vi "Build Dqmh Module Relationship Sub Graph.vi"(7 "Link Type":T1, 9 "Module Name":string, 10 "Links Info":T4[](array[typedef]), 11 "Graph in":refnum<class "Graph.lvclass">) -> (1 "Specific Edge Shape":T2[](array[typedef]), 2 "Specific Node Shape":T3[](array[typedef]), 3 "Graph out":refnum<class "Graph.lvclass">)   [LabVIEW 2021, in "TAF Proj Document Type.lvlib" / "Dqmh Module.lvclass"]
uses:
  <vilib>/Wovalab/AntiDoc/Document Type/Add-ons/LabVIEW TAF Project/Dqmh Module/Dqmh Module.lvclass
  <vilib>/Wovalab/AntiDoc/Document Type/Add-ons/LabVIEW TAF Project/Dqmh Module/Event Callers--cluster.ctl
  <vilib>/Wovalab/AntiDoc/GraphBuilder/Graph/Graph.lvclass
  <vilib>/Wovalab/AntiDoc/GraphBuilder/Renderer/Graphviz/Specific Node Shape Def.ctl
  <vilib>/Wovalab/AntiDoc/GraphBuilder/Shapes/Node/Graphviz/Graphviz Node Shape.lvclass
  <vilib>/Wovalab/AntiDoc/GraphBuilder/Renderer/Graphviz/Specific Edge Shape Def.ctl
  <vilib>/Wovalab/AntiDoc/GraphBuilder/Shapes/Edge/Graphviz/Graphviz Edge Shape.lvclass
  <vilib>/Wovalab/AntiDoc/Document Type/Add-ons/LabVIEW TAF Project/Dqmh Module/Link Type--enum.ctl
  <vilib>/Wovalab/AntiDoc/Document Type/Add-ons/LabVIEW TAF Project/Shared/Dqmh Event Module Link Type.ctl
  <vilib>/Wovalab/AntiDoc/Document Type/Add-ons/LabVIEW TAF Project/TAF Proj Document Type.lvlib
  <vilib>/Wovalab/AntiDoc/GraphBuilder/Renderer/Graphviz/Graphviz.lvclass
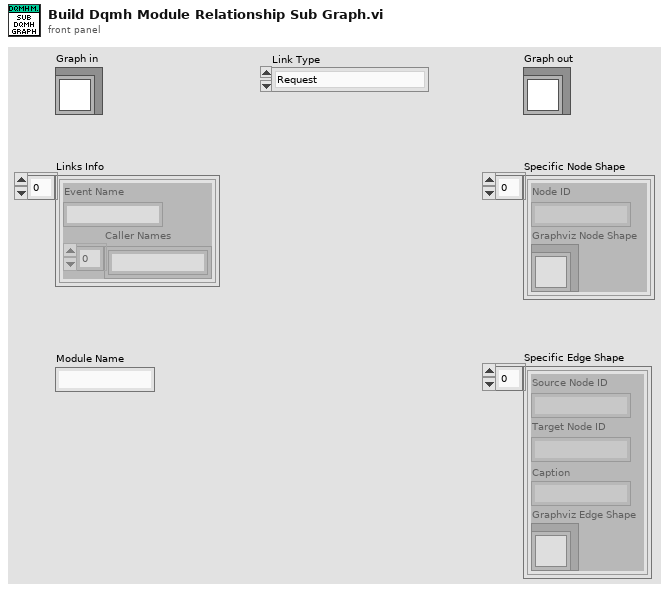
[diagram p1: front panel]
types:
  T1 = typedef "TAF Proj Document Type.lvlib/Dqmh Module.lvclass/Link Type--enum.ctl" = enum16{"Request", "Request With Reply", "Broadcast", "Registred Broadcast", "Used Requests", "Used Requests With Reply"}
  T2 = typedef "GraphBuilder.lvlib/Graphviz.lvclass/Specific Edge Shape Def.ctl" = cluster{"Source Node ID":string, "Target Node ID":string, "Caption":string, "Graphviz Edge Shape":refnum<class "Graphviz Edge Shape.lvclass">}
  T3 = typedef "GraphBuilder.lvlib/Graphviz.lvclass/Specific Node Shape Def.ctl" = cluster{"Node ID":string, "Graphviz Node Shape":refnum<class "Graphviz Node Shape.lvclass">}
  T4 = typedef "TAF Proj Document Type.lvlib/Dqmh Module.lvclass/Event Callers--cluster.ctl" = cluster{"Event Name":string, "Caller Names":string[]}
  T5 = typedef "TAF Proj Document Type.lvlib/Dqmh Event Module Link Type.ctl" = enum16{"Request", "Request With Reply", "Broadcast", "Registred Broadcast", "Used Requests", "Used Requests With Reply"}
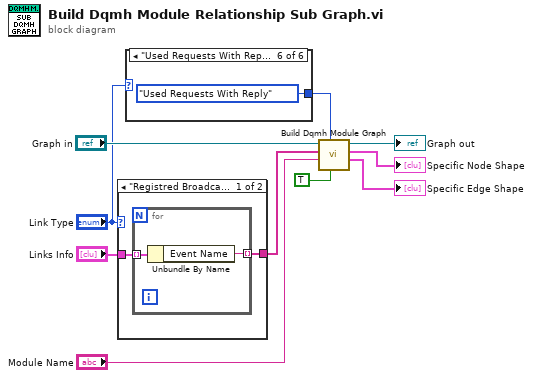
[diagram p0: block diagram]
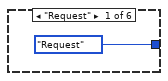
[diagram p2: hidden frame]
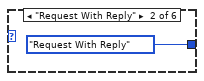
[diagram p3: hidden frame]
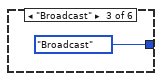
[diagram p4: hidden frame]
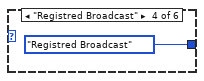
[diagram p5: hidden frame]
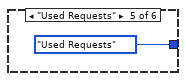
[diagram p6: hidden frame]
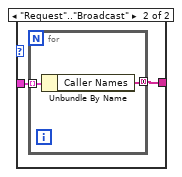
[diagram p7: hidden frame]
diagram:
  n1 = case shown="\"Registred Broadcast\"..\"Used Requests With Reply\"" "Link Type" {
    tunnel: "Links Info" -> [w12 w16]
    tunnel: [w11 w15] -> w8
    frame "Registred Broadcast".."Used Requests With Reply" {
      n2 = for {
        tunnel: w12 -> [w14] mode=indexing
        tunnel: [w13] -> w11 mode=indexing
        n3 = Unbundle By Name(w14) -> ("Event Name"=w13:string)
      }
    }
    frame "Request".."Broadcast" {
      n4 = for {
        tunnel: w16 -> [w18] mode=indexing
        tunnel: [w17] -> w15 mode=concatenating
        n5 = Unbundle By Name(w18) -> ("Caller Names"=w17:string[])
      }
    }
  }
  n6 = case shown="\"Used Requests With Reply\"" "Link Type" {
    tunnel: [Dqmh_Event_Module_Link_Type."Request" ("Link Type") Dqmh_Event_Module_Link_Type."Request With Reply" ("Link Type") Dqmh_Event_Module_Link_Type."Broadcast" ("Link Type") Dqmh_Event_Module_Link_Type."Registred Broadcast" ("Link Type") Dqmh_Event_Module_Link_Type."Used Requests" ("Link Type") Dqmh_Event_Module_Link_Type."Used Requests With Reply" ("Link Type")] -> w2
    frame "Request" {
    }
    frame "Request With Reply" {
    }
    frame "Broadcast" {
    }
    frame "Registred Broadcast" {
    }
    frame "Used Requests" {
    }
    frame "Used Requests With Reply" {
    }
  }
  n7 = call <vilib>:"Build Dqmh Module Graph.vi"("Draw API Tester Link"=TRUE, "Link Type"=w2, "Module Name"="Module Name", "Link Name"=w8, "Graph in"="Graph in") -> ("Specific Edge Shape"=→"Specific Edge Shape":T2[], "Specific Node Shape"=→"Specific Node Shape":T3[], "Graph out"=→"Graph out":refnum<class "Graph.lvclass">)  [unwired: 4 in]
